vi "Laser Power FGV.vi"(8 "error in (no error)":errorcluster, 10 "Laser Power":dbl, 11 "Action":T1) -> (0 "error out":errorcluster, 2 "Laser Power":dbl)   [LabVIEW 2022 SP3, in "Test Station SIM Laser Driver.lvclass"]
uses:
  Test Station SIM Laser Driver.lvclass
  Action.ctl
  Test Station SIM Laser Driver.lvclass/Test Station SIM Laser Driver.ctl
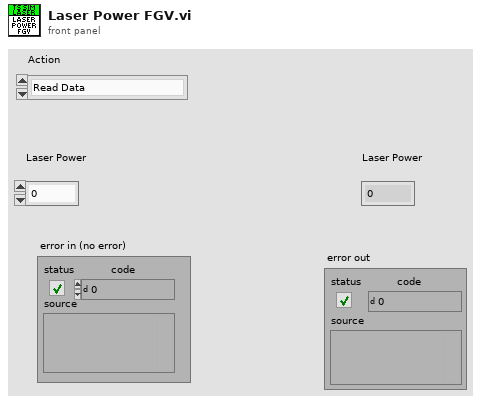
[diagram p1: front panel]
types:
  T1 = typedef "Test Station SIM Laser Driver.lvclass/Action.ctl" = enum16{"Read Data", "Set Data"}
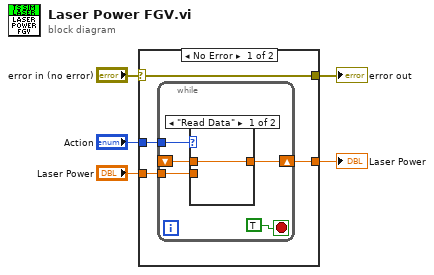
[diagram p0: block diagram]
diagram:
  n1 = case shown="No Error" "error in (no error)" {
    selector: "error in (no error)" -> [w6 w17]
    tunnel: "Action" -> [w9 _]
    tunnel: "Laser Power" -> [w8 _]
    tunnel: [w7 _] -> w1
    tunnel: [w6 w17] -> w2
    frame No Error {
      n2 = while {
        tunnel: w9 -> [w13]
        tunnel: w8 -> [w12]
        shift-right: [w11] -> w7
        shift-left: _ -> [w10]
        stop <- TRUE stop-if-true
        n3 = case shown="\"Read Data\"" w13 {
          tunnel: w12 -> [_ w16]
          tunnel: [w15 w16] -> w11
          tunnel: w10 -> [w15 _]
          frame "Read Data" {
          }
          frame "Set Data" {
          }
        }
      }
    }
    frame Error {
    }
  }
  "error out" <- w2
  "Laser Power" <- w1
